vi "Autonomous.vi"() -> ()   [LabVIEW 2017]
doc: "This VI starts when autonomous period begins, and will automatically be terminated when it ends. You can carry out timed or sensor driven operations directly to I/O or to subsystems without needing to return to the caller."
uses:
  Shared/PathFileData.ctl
  Shared/RobotNeededPathData.ctl
  Shared/AutoRoutineSelector.ctl
  53cd395b-8467-4eb9-a2a3-7883866f0301.vi
  <vilib>/Rock Robotics/Network Tables/NT Read Number.vi
  <vilib>/regexp/Match Regular Expression.xnode
  Shared/AutonomousRoutine.ctl
  64793a71-4a14-4a60-987c-f576e2f0ffc5.vi
  <vilib>/Rock Robotics/Network Tables/NT Read Numeric Array.vi
  <vilib>/Rock Robotics/Network Tables/NT Read Boolean.vi
  0e909f19-9ff0-427e-8bcb-a2de16ec1e77.vi
panel:
  out "File Path 4":string
  out "File Path 3":string
  out "PathData 2":T1
  in  "Path":T2
  in  "File Path 2":string="Test.txt"
  in  "Routine":i32
  out "File Path":string
  out "PathData":T1
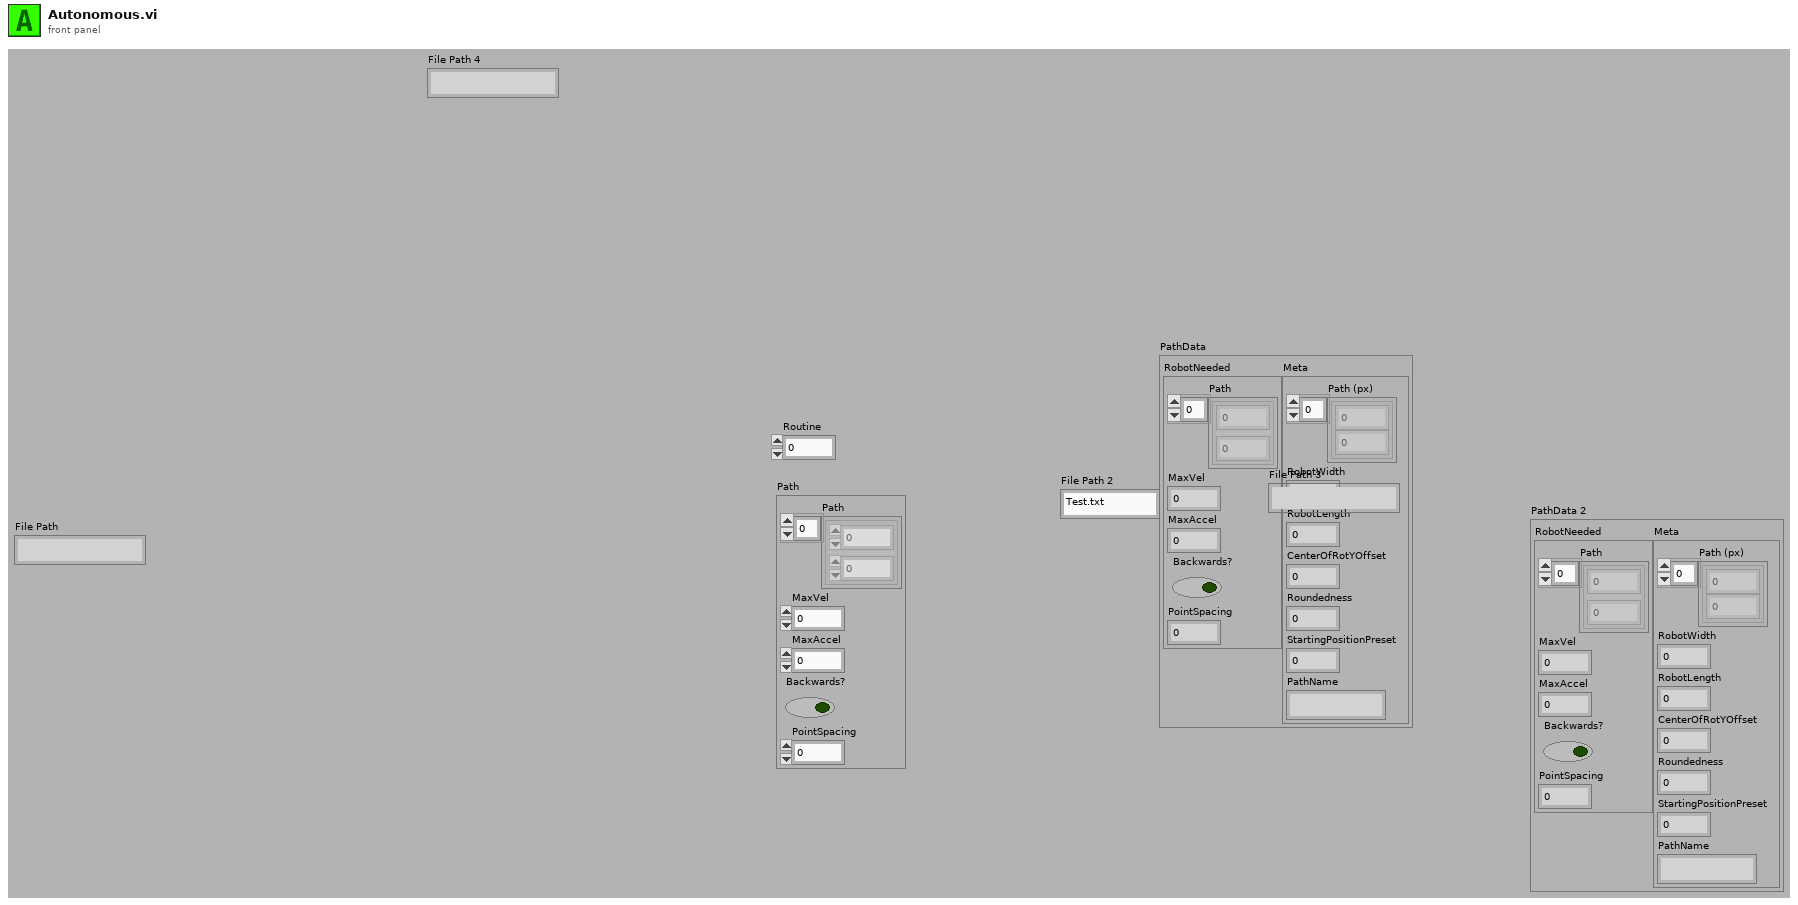
[diagram p1: front panel]
types:
  T1 = typedef "PathFileData.ctl" = cluster{"RobotNeeded":T2, "Meta":cluster{"Path (px)":cluster{i32, i32}[], "RobotWidth":dbl, "RobotLength":dbl, "CenterOfRotYOffset":dbl, "Roundedness":dbl, "StartingPositionPreset":u32, "PathName":string}}
  T2 = typedef "RobotNeededPathData.ctl" = cluster{"Path":cluster{dbl, dbl}[], "MaxVel":dbl, "MaxAccel":dbl, "Backwards?":bool, "PointSpacing":dbl}
  T3 = typedef "AutonomousRoutine.ctl" = enum16{"Score Scale", "Score Switch"}
  T4 = typedef "AutoRoutineSelector.ctl" = u16
  T5 = typedef "Command Status Info.ctl" = cluster{"Name":string, "Status":T6, "notifier out":T7}
  T6 = typedef "Completion Status.ctl" = enum16{"Successful", "Aborted", "Incomplete"}
  T7 = typedef "Completion Notifier.ctl" = refnum<notifier>
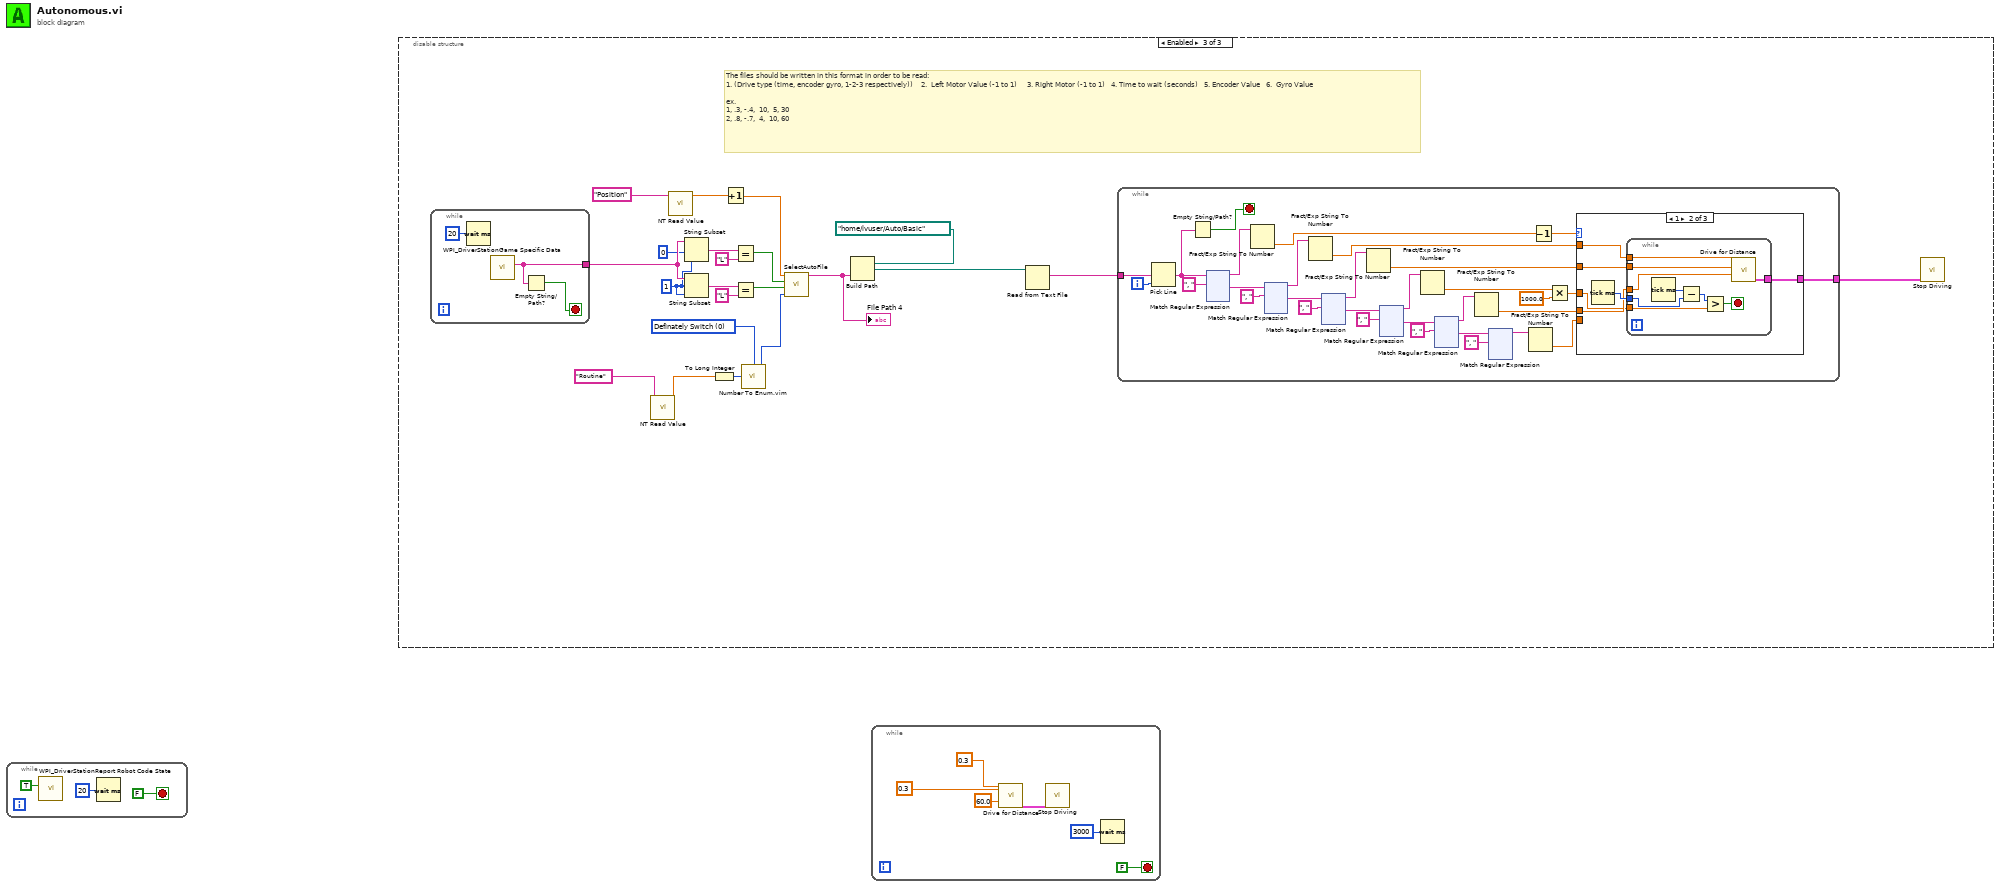
[diagram p0: block diagram]
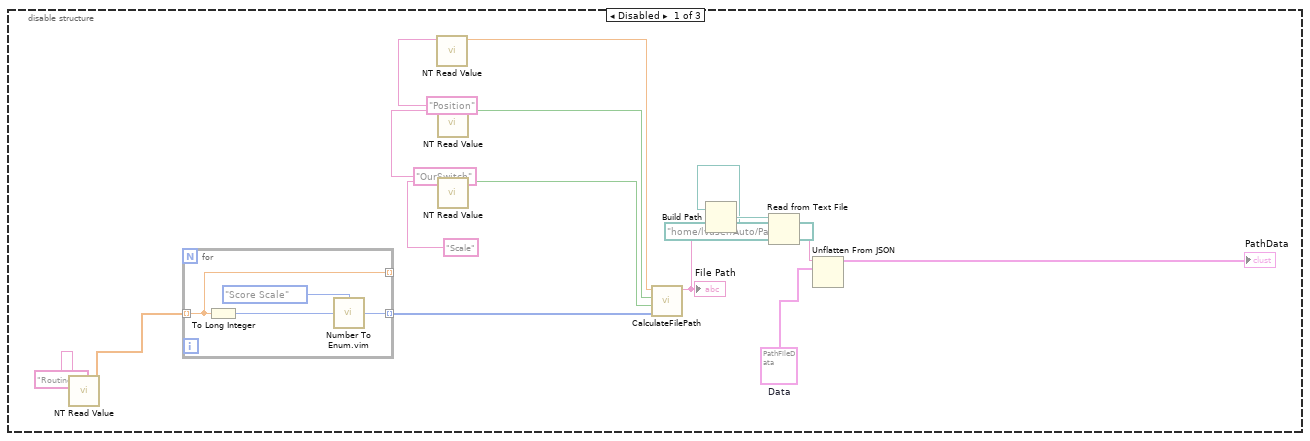
[diagram p2: hidden frame]
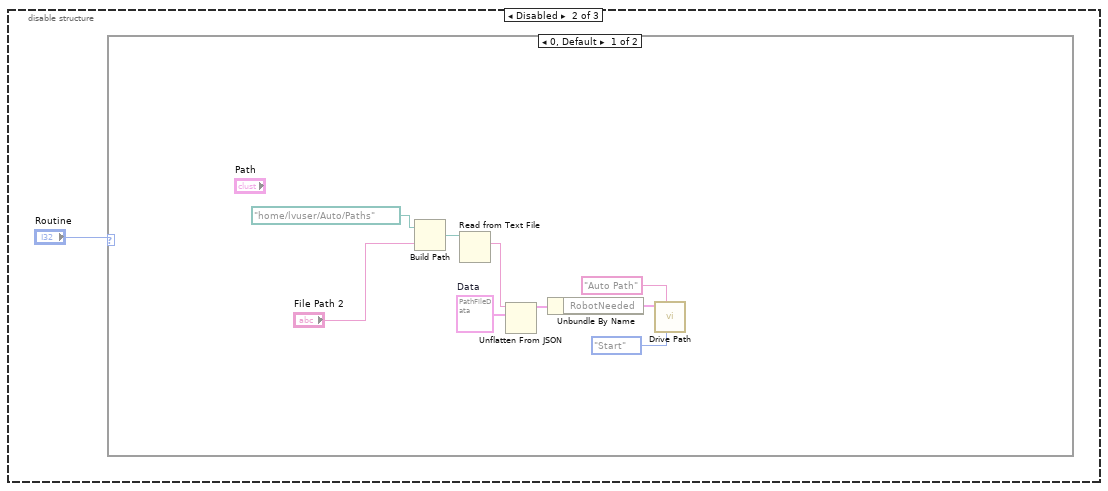
[diagram p3: hidden frame]
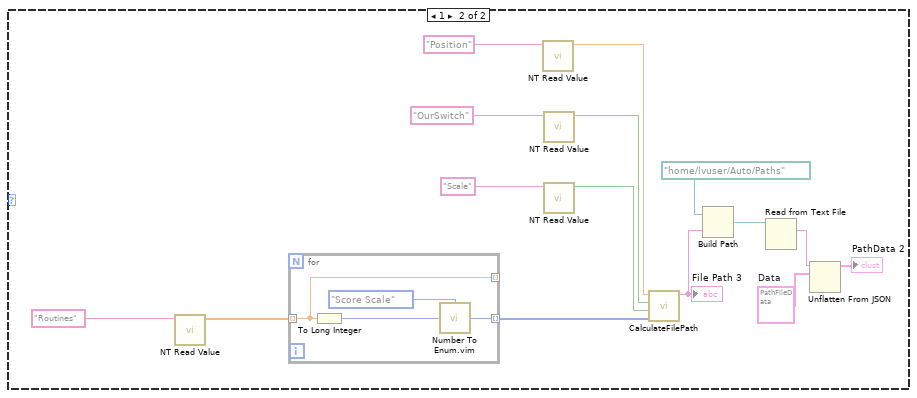
[diagram p4: hidden frame]
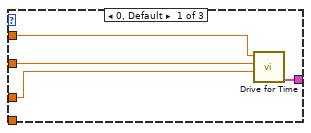
[diagram p5: hidden frame]
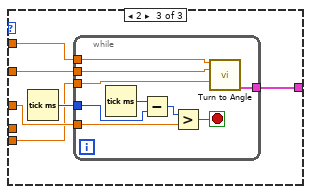
[diagram p6: hidden frame]
diagram:
  n1 = while {
    stop <- FALSE stop-if-true
    n2 = call <vilib>:"WPI_DriverStationReport Robot Code State.vi"("Autonomous"=TRUE) -> ()  [unwired: 10 in, 1 out]
    n3 = Wait (ms)(milliseconds to wait=u32 20) -> ()  [unwired: 1 out]
  }
  n4 = disable-structure shown="Enabled" {
    frame Disabled {
      w4 = T1 {"RobotNeeded"={"Path"=[], "MaxVel"=0.0, "MaxAccel"=0.0, "Backwards?"=FALSE, "PointSpacing"=0.0}, "Meta"={"Path (px)"=[], "RobotWidth"=0.0, "RobotLength"=0.0, "CenterOfRotYOffset"=0.0, "Roundedness"=0.0, "StartingPositionPreset"=0, "PathName"=""}}  # Data
      n5 = call-poly <vilib>:"NT Read Value.vi"("Name"="Routines") -> ("Numeric Array"=w14:dbl[])  [unwired: 9 in, 1 out]
      n6 = for {
        tunnel: w14 -> [w20] mode=indexing
        tunnel: [w20] -> _ mode=indexing
        tunnel: [w22] -> w15 mode=indexing
        n7 = To Long Integer(number=w20) -> (32bit integer=w21:i32)
        n8 = call "Number To Enum.vim"("number"=w21, "enum type"=AutonomousRoutine."Score Scale" ("LL")) -> ("number as enum"=w22:T3)
      }
      n9 = call-poly <vilib>:"NT Read Value.vi"("Name"="Position") -> ("Numeric"=w18:dbl)  [unwired: 9 in, 1 out]
      n10 = call-poly <vilib>:"NT Read Value.vi"("Name"="OurSwitch") -> ("Boolean"=w10:bool)  [unwired: 9 in, 1 out]
      n11 = call-poly <vilib>:"NT Read Value.vi"("Name"="Scale") -> ("Boolean"=w12:bool)  [unwired: 9 in, 1 out]
      n12 = call "CalculateFilePath.vi"("Routines"=w15, "Scale"=w12, "OurSwitch"=w10, "Position"=w18) -> ("File Name"=w16:string)  [unwired: 7 in]
      "File Path" <- w16
      n13 = Build Path(base path=path "/home/lvuser/Auto/Paths", name or relative path=w16) -> (appended path=w8:path)
      n14 = Read from Text File(file (use dialog)=w8) -> (text=w6:string)  [unwired: 3 in, 3 out]
      n15 = Unflatten From JSON(JSON string=w6, type and defaults=w4) -> (value=→"PathData":T1)  [unwired: 5 in, 1 out]
    }
    frame Disabled {
      n16 = case shown="0, Default" "Routine" {
        frame 0, Default {
          w27 = T1 {"RobotNeeded"={"Path"=[], "MaxVel"=0.0, "MaxAccel"=0.0, "Backwards?"=FALSE, "PointSpacing"=0.0}, "Meta"={"Path (px)"=[], "RobotWidth"=0.0, "RobotLength"=0.0, "CenterOfRotYOffset"=0.0, "Roundedness"=0.0, "StartingPositionPreset"=0, "PathName"=""}}  # Data
          n17 = Build Path(base path=path "/home/lvuser/Auto/Paths", name or relative path="File Path 2") -> (appended path=w31:path)
          n18 = Read from Text File(file (use dialog)=w31) -> (text=w30:string)  [unwired: 3 in, 3 out]
          n19 = Unflatten From JSON(JSON string=w30, type and defaults=w27) -> (value=w26:T1)  [unwired: 5 in, 1 out]
          n20 = Unbundle By Name(w26) -> ("RobotNeeded"=w25:T2)
          n21 = call "Drive Path.vi"("Synchronication"=enum16{"Start", "Wait"}."Start", "Description"="Auto Path", "Path"=w25) -> ()  [unwired: 8 in, 1 out]
        }
        frame 1 {
          w33 = T1 {"RobotNeeded"={"Path"=[], "MaxVel"=0.0, "MaxAccel"=0.0, "Backwards?"=FALSE, "PointSpacing"=0.0}, "Meta"={"Path (px)"=[], "RobotWidth"=0.0, "RobotLength"=0.0, "CenterOfRotYOffset"=0.0, "Roundedness"=0.0, "StartingPositionPreset"=0, "PathName"=""}}  # Data
          n22 = call-poly <vilib>:"NT Read Value.vi"("Name"="Routines") -> ("Numeric Array"=w43:dbl[])  [unwired: 9 in, 1 out]
          n23 = for {
            tunnel: w43 -> [w49] mode=indexing
            tunnel: [w49] -> _ mode=indexing
            tunnel: [w51] -> w44 mode=indexing
            n24 = To Long Integer(number=w49) -> (32bit integer=w50:i32)
            n25 = call "Number To Enum.vim"("number"=w50, "enum type"=AutonomousRoutine."Score Scale" ("LL")) -> ("number as enum"=w51:T3)
          }
          n26 = call-poly <vilib>:"NT Read Value.vi"("Name"="Position") -> ("Numeric"=w47:dbl)  [unwired: 9 in, 1 out]
          n27 = call-poly <vilib>:"NT Read Value.vi"("Name"="OurSwitch") -> ("Boolean"=w39:bool)  [unwired: 9 in, 1 out]
          n28 = call-poly <vilib>:"NT Read Value.vi"("Name"="Scale") -> ("Boolean"=w41:bool)  [unwired: 9 in, 1 out]
          n29 = call "CalculateFilePath.vi"("Routines"=w44, "Scale"=w41, "OurSwitch"=w39, "Position"=w47) -> ("File Name"=w45:string)  [unwired: 7 in]
          "File Path 3" <- w45
          n30 = Build Path(base path=path "/home/lvuser/Auto/Paths", name or relative path=w45) -> (appended path=w37:path)
          n31 = Read from Text File(file (use dialog)=w37) -> (text=w35:string)  [unwired: 3 in, 3 out]
          n32 = Unflatten From JSON(JSON string=w35, type and defaults=w33) -> (value=→"PathData 2":T1)  [unwired: 5 in, 1 out]
        }
      }
    }
    frame Enabled {
      w54 = T4 0 items=["Definately Switch", "Definately Scale", "Switch if in front, else scale", "Scale if in front, else switch", "Switch if in front, else nothing", "Scale if in front, else nothing", "Drive across line"] ("Routine")
      w58 = 1 ("length (rest)")
      # "The files should be written in this format in order to be read:\n1. (Drive type (time, encoder gyro, 1-2-3 respectively))    2.  Left Motor Value (-1 to 1)     3. Right Motor (-1 to 1)   4. Time to wait (seconds)   5. Encoder Value   6.  Gyro Value\n\nex. \n1, .3, -.4,  10,  5, 30\n2, .8, -.7,  4,  10, 60"
      n33 = while {
        tunnel: [w76] -> w71
        stop <- w75 stop-if-true
        n34 = Wait (ms)(milliseconds to wait=u32 20) -> ()  [unwired: 1 out]
        n35 = call <vilib>:"WPI_DriverStationGame Specific Data.vi"() -> ("Game Specific Data"=w76:string)  [unwired: 11 in]
        n36 = Empty String/Path?(string/path=w76) -> (empty?=w75:bool)
      }
      n37 = call-poly <vilib>:"NT Read Value.vi"("Name"="Routine") -> ("Numeric"=w70:dbl)  [unwired: 9 in, 1 out]
      n38 = call-poly <vilib>:"NT Read Value.vi"("Name"="Position") -> ("Numeric"=w72:dbl)  [unwired: 9 in, 1 out]
      n39 = String Subset(string=w71, offset (0)=0 ("length (rest)"), length (rest)=w58) -> (substring=w69:string)
      n40 = String Subset(string=w71, offset (0)=w58, length (rest)=w58) -> (substring=w68:string)
      n41 = To Long Integer(number=w70) -> (32bit integer=w67:i32)
      n42 = Increment(x=w72) -> (x+1=w66:dbl)
      n43 = Equal?(x=w69, y="L") -> (x = y?=w65:bool)
      n44 = Equal?(x=w68, y="L") -> (x = y?=w64:bool)
      n45 = call "Number To Enum.vim"("number"=w67, "enum type"=w54) -> ("number as enum"=w63:T4)
      n46 = call "SelectAutoFile.vi"("Routine"=w63, "OurSwitch"=w64, "OurScale"=w65, "Position"=w66) -> ("File Name"=w73:string)  [unwired: 7 in]
      "File Path 4" <- w73
      n47 = Build Path(base path=path "/home/lvuser/Auto/Basic", name or relative path=w73) -> (appended path=w62:path)
      n48 = Read from Text File(file (use dialog)=w62) -> (text=w61:string)  [unwired: 3 in, 3 out]
      n49 = while {
        tunnel: w61 -> [w106]
        tunnel: [w77] -> w52
        i -> [w107]
        stop <- w105 stop-if-true
        n50 = Pick Line(multi-line string=w106, line index=w107) -> (output string=w103:string)  [unwired: 1 in]
        n51 = Empty String/Path?(string/path=w103) -> (empty?=w105:bool)
        n52 = xnode "Match Regular Expression"("input string"=w103, "regular expression"=", ") -> ("before match"=w104:string, "after match"=w99:string)  [unwired: 4 in, 3 out]
        n53 = Fract/Exp String To Number(string=w104) -> (number=w101:dbl)  [unwired: 3 in, 1 out]
        n54 = xnode "Match Regular Expression"("input string"=w99, "regular expression"=", ") -> ("before match"=w90:string, "after match"=w91:string)  [unwired: 4 in, 3 out]
        n55 = Fract/Exp String To Number(string=w90) -> (number=w82:dbl)  [unwired: 3 in, 1 out]
        n56 = xnode "Match Regular Expression"("input string"=w91, "regular expression"=", ") -> ("before match"=w92:string, "after match"=w93:string)  [unwired: 4 in, 3 out]
        n57 = Fract/Exp String To Number(string=w92) -> (number=w81:dbl)  [unwired: 3 in, 1 out]
        n58 = xnode "Match Regular Expression"("input string"=w93, "regular expression"=", ") -> ("before match"=w94:string, "after match"=w95:string)  [unwired: 4 in, 3 out]
        n59 = Fract/Exp String To Number(string=w94) -> (number=w83:dbl)  [unwired: 3 in, 1 out]
        n60 = xnode "Match Regular Expression"("input string"=w95, "regular expression"=", ") -> ("before match"=w96:string, "after match"=w97:string)  [unwired: 4 in, 3 out]
        n61 = Fract/Exp String To Number(string=w96) -> (number=w79:dbl)  [unwired: 3 in, 1 out]
        n62 = xnode "Match Regular Expression"("input string"=w97, "regular expression"=", ") -> ("before match"=w98:string)  [unwired: 4 in, 4 out]
        n63 = Fract/Exp String To Number(string=w98) -> (number=w78:dbl)  [unwired: 3 in, 1 out]
        n64 = Decrement(x=w101) -> (x-1=w100:dbl)
        n65 = Multiply(x=w83, y=1000.0) -> (x*y=w80:dbl)
        n66 = case shown="1" w100 {
          tunnel: w82 -> [w681 w686 w700]
          tunnel: w81 -> [w680 w685 w699]
          tunnel: w80 -> [w679 w683 w701]
          tunnel: w79 -> [_ w684 _]
          tunnel: w78 -> [_ _ w698]
          tunnel: [w678 w682 w697] -> w77
          frame 0, Default {
            n67 = call "Drive for Time.vi"("Seconds"=w679, "Right Speed"=w680, "Left Speed"=w681) -> ("Command Info Out"=w678:T5)  [unwired: 7 in, 1 out]
          }
          frame 1 {
            n68 = Tick Count (ms)() -> (millisecond timer value=w687:u32)
            n69 = while {
              tunnel: w687 -> [w696]
              tunnel: w683 -> [w693]
              tunnel: w686 -> [w691]
              tunnel: w685 -> [w690]
              tunnel: w684 -> [w689]
              tunnel: [w688] -> w682
              stop <- w692 stop-if-true
              n70 = Tick Count (ms)() -> (millisecond timer value=w695:u32)
              n71 = Subtract(x=w695, y=w696) -> (x-y=w694:u32)
              n72 = Greater?(x=w694, y=w693) -> (0:w692:bool)
              n73 = call "Drive for Distance.vi"("Left Setpoint"=w691, "Right Setpoint"=w690, "Distance"=w689) -> ("Command Info Out"=w688:T5)  [unwired: 12 in]
            }
          }
          frame 2 {
            n74 = Tick Count (ms)() -> (millisecond timer value=w702:u32)
            n75 = while {
              tunnel: w702 -> [w711]
              tunnel: w701 -> [w708]
              tunnel: w700 -> [w706]
              tunnel: w699 -> [w705]
              tunnel: w698 -> [w704]
              tunnel: [w703] -> w697
              stop <- w707 stop-if-true
              n76 = Tick Count (ms)() -> (millisecond timer value=w710:u32)
              n77 = Subtract(x=w710, y=w711) -> (x-y=w709:u32)
              n78 = Greater?(x=w709, y=w708) -> (0:w707:bool)
              n79 = call "Turn to Angle.vi"("Left Speed"=w706, "Right Speed"=w705, "Angle"=w704) -> ("Command Info Out"=w703:T5)  [unwired: 12 in]
            }
          }
        }
      }
      n80 = call "Stop Driving.vi"("Command Info In"=w52) -> ()  [unwired: 10 in, 1 out]
    }
  }
  n81 = while {
    stop <- FALSE stop-if-true
    n82 = call "Drive for Distance.vi"("Left Setpoint"=0.3, "Right Setpoint"=0.3, "Distance"=60.0) -> ("Command Info Out"=w828:T5)  [unwired: 12 in]
    n83 = call "Stop Driving.vi"("Command Info In"=w828) -> ()  [unwired: 10 in, 1 out]
    n84 = Wait (ms)(milliseconds to wait=u32 3000) -> ()  [unwired: 1 out]
  }
